vi "Test MQTT-3.1.3-7.vi"(8 "error in (no error)":errorcluster) -> (0 "error out":errorcluster)   [LabVIEW 2013]
uses:
  source/Control Packets/CONNACK/Connect Return Code -- enum.ctl
  source/Control Packets/CONNECT/ConnectFlags -- cluster.ctl
  <vilib>/addons/_JKI Toolkits/Caraya/classes/Test/Test.lvclass
  source/Control Packets/CONNACK/CONNACK.lvclass
  <vilib>/addons/_JKI Toolkits/Caraya/classes/Assert/Assert.lvclass
  source/Client/Client.lvclass
  source/Control Packets/CONNECT/CONNECT.lvclass
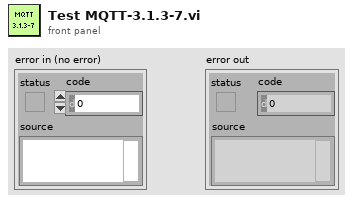
[diagram p1: front panel]
types:
  T1 = typedef "CONNECT.lvclass/ConnectFlags -- cluster.ctl" = cluster{"Reserved":bool, "Clean Session":bool, "Will Flag":bool, "Will QoS 1":bool, "Will QoS 2":bool, "Will Retain":bool, "Password Flag":bool, "User Name Flag":bool}
  T2 = typedef "CONNACK.lvclass/Connect Return Code -- enum.ctl" = enum16{"Connection accepted", "Unacceptable protocol version", "Identifier Rejected", "Server Unavailable", "Bad Username or Password", "Not Authorized"}
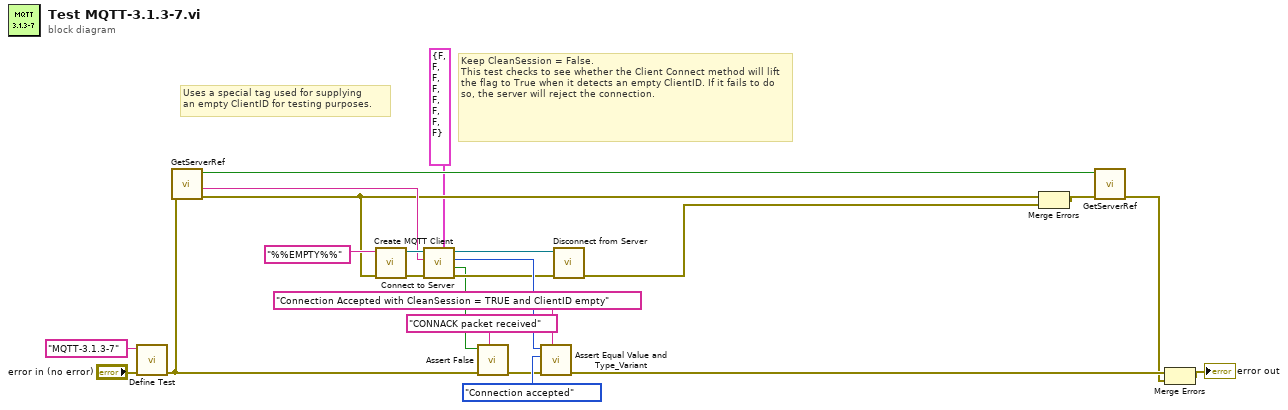
[diagram p0: block diagram]
diagram:
  # "Keep CleanSession = False.\nThis test checks to see whether the Client Connect method will lift the flag to True when it detects an empty ClientID. If it fails to do so, the server will reject the connection."
  # "Uses a special tag used for supplying\nan empty ClientID for testing purposes."
  n1 = call <vilib>:"Define Test.vi"("error in (no error)"="error in (no error)", "Label (VI Title)"="MQTT-3.1.3-7") -> ("error out"=w3:errorcluster)  [unwired: 9 in]
  n2 = call "GetServerRef.vi"("error in"=w3) -> ("error out"=w2:errorcluster, "Server address"=w4:string, "Created"=w15:bool)  [unwired: 7 in, 1 out]
  n3 = call "Create MQTT Client.vi"("error in (no error)"=w2, "ID (empty:generate new)"="%%EMPTY%%" ("Client ID (empty: generate new)")) -> ("error out"=w10:errorcluster, "Client out"=w11:refnum<class "Client.lvclass">)  [unwired: 8 in]
  n4 = call "Connect to Server.vi"("Connect Flags"=T1 {"Reserved"=FALSE, "Clean Session"=FALSE, "Will Flag"=FALSE, "Will QoS 1"=FALSE, "Will QoS 2"=FALSE, "Will Retain"=FALSE, "Password Flag"=FALSE, "User Name Flag"=FALSE}, "error in (no error)"=w10, "address (localhost)"=w4, "Client in"=w11) -> ("error out"=w7:errorcluster, "timed out"=w6:bool, "Return Code"=w9:T2, "Client out"=w8:refnum<class "Client.lvclass">)  [unwired: 4 in]
  n5 = call <vilib>:"Assert False.vi"("Label"="CONNACK packet received", "error in (no error)"=w3, "False?"=w6) -> ("error out"=w17:errorcluster)  [unwired: 8 in]
  n6 = call <vilib>:"Assert Equal Value and Type_Variant.vi"("Label"="Connection Accepted with CleanSession = TRUE and ClientID empty", "error in (no error)"=w17, "Y"=Connect_Return_Code_--_enum."Connection accepted" ("Return Code"), "X"=w9) -> ("error out"=w22:errorcluster)  [unwired: 7 in]
  n7 = call "Disconnect from Server.vi"("error in (no error)"=w7, "Client in"=w8) -> ("error out"=w5:errorcluster)  [unwired: 7 in, 2 out]
  n8 = Merge Errors(w2, w5) -> (w14:errorcluster)
  n9 = call "GetServerRef.vi"("error in"=w14, "Destroy (F)"=w15) -> ("error out"=w13:errorcluster)  [unwired: 6 in, 3 out]
  n10 = Merge Errors(w22, w13) -> (→"error out":errorcluster)
